vi "Catch.vi"(7 "Action":T1=enum."Stop", 8 "error in (no error)":errorcluster) -> (0 "error out":errorcluster)   [LabVIEW 2013]
uses:
  CatchEnum.ctl
  DoubleSolenoidAction.ctl
  RollerAction.ctl
  SingleSolenoidAction.ctl
  PnuematicMode.ctl
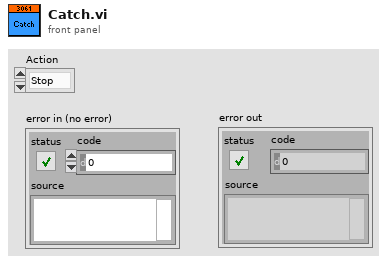
[diagram p1: front panel]
types:
  T1 = typedef "CatchEnum.ctl" = enum16{"PreCatch", "Catch", "Stop"}
  T2 = typedef "SingleSolenoidAction.ctl" = enum16{"Init", "SetState", "Disable"}
  T3 = typedef "RollerAction.ctl" = enum16{"Init", "Off", "Forward", "Reverse"}
  T4 = typedef "DoubleSolenoidAction.ctl" = enum16{"Init", "Middle", "In", "Out"}
  T5 = typedef "PnuematicMode.ctl" = enum16{"Init", "SetState", "Disable"}
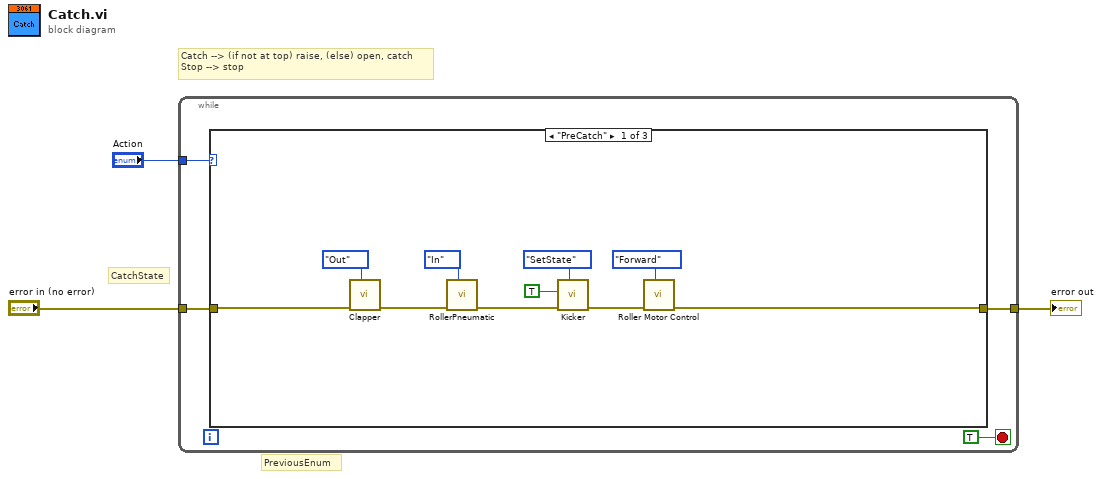
[diagram p0: block diagram]
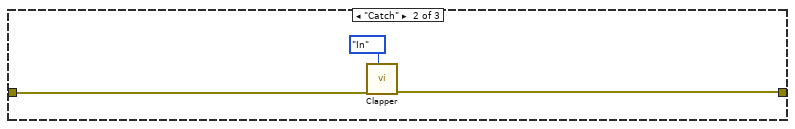
[diagram p2: hidden frame]
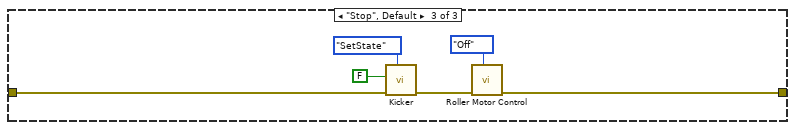
[diagram p3: hidden frame]
diagram:
  # "CatchState"
  # "Catch --> (if not at top) raise, (else) open, catch\nStop --> stop"
  # "PreviousEnum"
  n1 = while {
    tunnel: "error in (no error)" -> [w7]
    tunnel: [w6] -> w2
    tunnel: "Action" -> [w5]
    stop <- TRUE stop-if-true
    n2 = case shown="\"PreCatch\"" w5 {
      tunnel: w7 -> [w12 w19 w21]
      tunnel: [w10 w18 w23] -> w6
      frame "PreCatch" {
        n3 = call "Clapper.vi"("State"=DoubleSolenoidAction."Out", "Error in"=w12) -> ("Error out"=w13:errorcluster)  [unwired: 9 in]
        n4 = call "RollerPneumatic.vi"("State"=DoubleSolenoidAction."In", "Error in"=w13) -> ("Error out"=w14:errorcluster)  [unwired: 9 in]
        n5 = call "Kicker.vi"("Action"=SingleSolenoidAction."SetState", "error in (no error)"=w14, "Actuate?"=TRUE) -> ("error out"=w11:errorcluster)  [unwired: 8 in]
        n6 = call "Roller Motor Control.vi"("Action"=RollerAction."Forward", "Error in"=w11) -> ("Error out"=w10:errorcluster)  [unwired: 9 in]
      }
      frame "Catch" {
        n7 = call "Clapper.vi"("State"=DoubleSolenoidAction."In", "Error in"=w19) -> ("Error out"=w18:errorcluster)  [unwired: 9 in]
      }
      frame "Stop", Default {
        n8 = call "Kicker.vi"("Action"=PnuematicMode."SetState" ("Mode"), "error in (no error)"=w21, "Actuate?"=FALSE) -> ("error out"=w24:errorcluster)  [unwired: 8 in]
        n9 = call "Roller Motor Control.vi"("Action"=RollerAction."Off", "Error in"=w24) -> ("Error out"=w23:errorcluster)  [unwired: 9 in]
      }
    }
  }
  "error out" <- w2
